vi "getWorldProperties_parse.vi"(8 "error in":errorcluster, 11 "msg in":string) -> (0 "error out":errorcluster, 2 "WorldProperties":T1, 3 "msg out":string)   [LabVIEW 2012]
uses:
  <userlib>/rosforlv/ROS/parsing/std_msgs/subs/parse_u8_scalar.vi
  <userlib>/rosforlv/ROS/parsing/std_msgs/subs/parse_float64_scalar.vi
  <userlib>/rosforlv/ROS/parsing/std_msgs/subs/parse_string_array.vi
  <userlib>/rosforlv/ROS/parsing/std_msgs/subs/parse_bool_scalar.vi
  <userlib>/rosforlv/ROS/parsing/std_msgs/subs/parse_string_scalar.vi
panel:
  out "error byte":u8
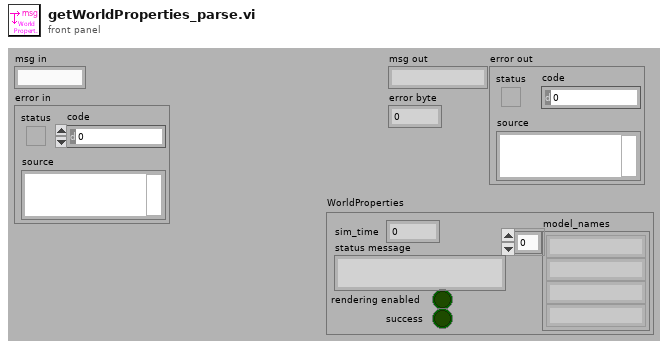
[diagram p1: front panel]
types:
  T1 = cluster{"sim_time":dbl, "model_names":string[], "rendering enabled":bool, "success":bool, "status message":string}
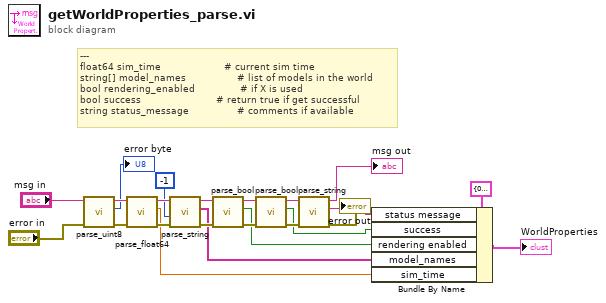
[diagram p0: block diagram]
diagram:
  # "---\nfloat64 sim_time                     # current sim time\nstring[] model_names                 # list of models in the world\nbool rendering_enabled               # if X is used\nbool success                         # return true if get successful\nstring status_message                # comments if available"
  n1 = call-poly <userlib>:"parse_uint8.vi"("error in"="error in", "msg in"="msg in") -> ("error out"=w2:errorcluster, "number"=→"error byte":u8, "msg out"=w3:string)  [unwired: 3 in]
  n2 = call-poly <userlib>:"parse_float64.vi"("error in"=w2, "msg in"=w3) -> ("error out"=w23:errorcluster, "number"=w11:dbl, "msg out"=w22:string)  [unwired: 3 in]
  n3 = call-poly <userlib>:"parse_string.vi"("error in"=w23, "Array Size"=-1, "msg in"=w22) -> ("error out"=w20:errorcluster, "strings"=w10:string[], "msg out"=w21:string)  [unwired: 2 in]
  n4 = call-poly <userlib>:"parse_bool.vi"("error in"=w20, "msg in"=w21) -> ("error out"=w19:errorcluster, "bool"=w9:bool, "msg out"=w18:string)  [unwired: 3 in]
  n5 = call-poly <userlib>:"parse_bool.vi"("error in"=w19, "msg in"=w18) -> ("error out"=w17:errorcluster, "bool"=w8:bool, "msg out"=w16:string)  [unwired: 3 in]
  n6 = call-poly <userlib>:"parse_string.vi"("error in"=w17, "msg in"=w16) -> ("error out"=→"error out":errorcluster, "string"=w7:string, "msg out"=→"msg out":string)  [unwired: 3 in]
  n7 = Bundle By Name(cluster=T1 {"sim_time"=0.0, "model_names"=[], "rendering enabled"=FALSE, "success"=FALSE, "status message"=""} ("GetWorldProperties"), "status message"=w7, "success"=w8, "rendering enabled"=w9, "model_names"=w10, "sim_time"=w11) -> (→"WorldProperties":T1)
